vi "Create_Trajectory_Get_RectRegion_Constraint.vi"(11 "inTRAJECTORY_CONFIG":T1 {"End Velocity" format="%20.4f"; "StartVelocity" format="%20.4f"; "Max Acceleration" format="%20.4f"; "MaxVelocity" format="%20.4f"}) -> (1 "Constraint Exists":bool, 3 "Rect Region Constraint":T2={"BottomLeftPoint"={"X"=0.0, "Y"=0.0}, "TopRightPoint"={"X"=0.0, "Y"=0.0}, "Constraint"=variant, "Constraint Type"=enum."DIFF DRIVE KINEMATICS"} {"TopRightPoint"."Y" format="%14.3f"; "TopRightPoint"."X" format="%14.3f"; "BottomLeftPoint"."Y" format="%14.3f"; "BottomLeftPoint"."X" format="%14.3f"})   [LabVIEW 2019]
doc: "Retrieves the Differntial Drive Kinematics constraint from the Trajectory Configuration.\n\nNote: If more than once instance of the Differntial Drive Kinematics constraint exists only the first one is returned. (Only one of these should be defined.)\n\nParameters:\n - InTrajectoryConfig -- The trajectory configuration data structure\n\nReturns:\n - Diff Drive Kinematics Constraint -- The data cluster, which contains the constraint.\n - Constraint Exists -- Returns TRUE if this constraint is defined in the trjaectory configuration."
uses:
  <vilib>/Rock Robotics/WPI/ThirdParty/JAS_Junk/TrajLib/TypeDef/TRAJ_CONSTRAINT_RECT_REGION.ctl
  <vilib>/Rock Robotics/WPI/ThirdParty/JAS_Junk/TrajLib/TypeDef/TRANSLATION2D.ctl
  <vilib>/Rock Robotics/WPI/ThirdParty/JAS_Junk/TrajLib/Enum/TRAJ_CONSTRAINT_TYPES_ENUM.ctl
  <vilib>/Rock Robotics/WPI/ThirdParty/JAS_Junk/TrajLib/TypeDef/TRAJ_CONFIG.ctl
  <vilib>/Utility/Data Type/NI_Data Type.lvlib
  <vilib>/Rock Robotics/WPI/ThirdParty/JAS_Junk/TrajLib/Trajectory_Library.lvlib
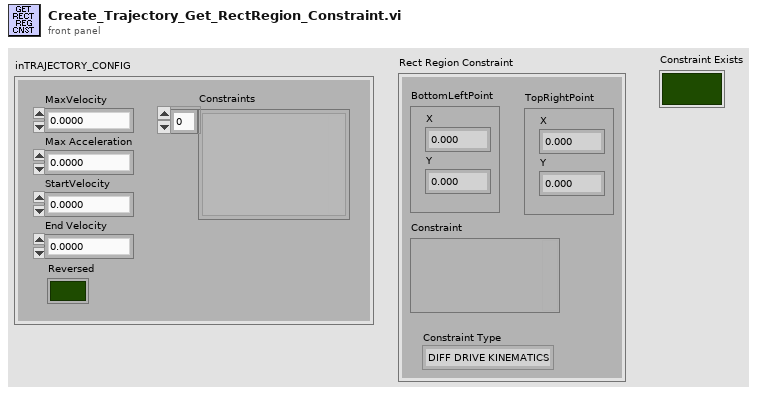
[diagram p1: front panel]
types:
  T1 = typedef "Trajectory_Library.lvlib/TRAJ_CONFIG.ctl" = cluster{"MaxVelocity":dbl, "Max Acceleration":dbl, "StartVelocity":dbl, "End Velocity":dbl, "Reversed":bool, "Constraints":variant[]}
  T2 = typedef "Trajectory_Library.lvlib/TRAJ_CONSTRAINT_RECT_REGION.ctl" = cluster{"BottomLeftPoint":T3, "TopRightPoint":T3, "Constraint":variant, "Constraint Type":T4}
  T3 = typedef "Trajectory_Library.lvlib/TRANSLATION2D.ctl" = cluster{"X":dbl, "Y":dbl}
  T4 = typedef "Trajectory_Library.lvlib/TRAJ_CONSTRAINT_TYPES_ENUM.ctl" = enum16{"UNDEFINED", "DIFF DRIVE KINEMATICS", "DIFF DRIVE VOLTAGE", "CENTRIPITAL ACCEL", "MECA DRIVE KINEMATICS", "SWERVE DRIVE KINEMATICS", "MAXIMUM VELOCITY", "ELLIPTICAL REGION", "RECTANGULAR REGION"}
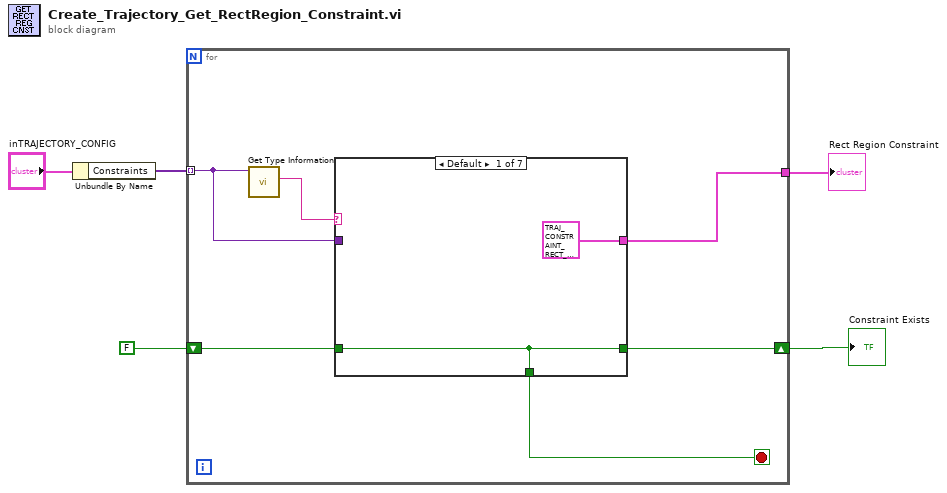
[diagram p0: block diagram]
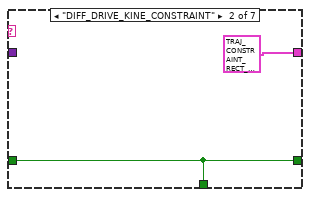
[diagram p2: hidden frame]
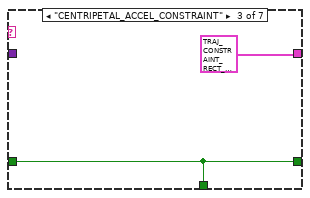
[diagram p3: hidden frame]
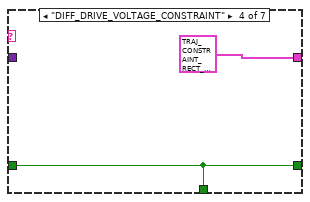
[diagram p4: hidden frame]
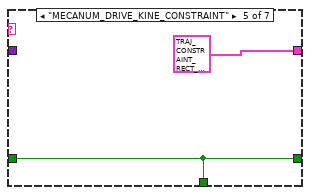
[diagram p5: hidden frame]
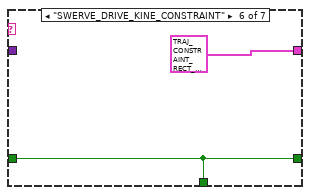
[diagram p6: hidden frame]
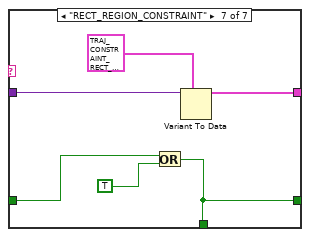
[diagram p7: hidden frame]
diagram:
  n1 = Unbundle By Name("inTRAJECTORY_CONFIG") -> ("Constraints"=w4:variant[])
  n2 = for {
    tunnel: w4 -> [w10] mode=indexing
    shift-right: [w8] -> w2
    shift-left: FALSE -> [w9]
    tunnel: [w6] -> w1
    stop <- w7 stop-if-true
    n3 = call <vilib>:"Get Type Information.vi"("variant"=w10) -> ("name"=w11:string)  [unwired: 6 in, 4 out]
    n4 = case shown="Default" w11 {
      tunnel: w10 -> [_ _ _ _ _ _ w25]
      tunnel: w9 -> [w13 w14 w17 w19 w21 w23 w28]
      tunnel: [w13 w14 w17 w19 w21 w23 w27] -> w8
      tunnel: [w13 w14 w17 w19 w21 w23 w27] -> w7
      tunnel: [T2 {"BottomLeftPoint"={"X"=0.0, "Y"=0.0}, "TopRightPoint"={"X"=0.0, "Y"=0.0}, "Constraint"=variant, "Constraint Type"=enum."DIFF DRIVE KINEMATICS"} ("Diff Drive Kinematics Constraint 2") T2 {"BottomLeftPoint"={"X"=0.0, "Y"=0.0}, "TopRightPoint"={"X"=0.0, "Y"=0.0}, "Constraint"=variant, "Constraint Type"=enum."DIFF DRIVE KINEMATICS"} ("Diff Drive Kinematics Constraint 2") T2 {"BottomLeftPoint"={"X"=0.0, "Y"=0.0}, "TopRightPoint"={"X"=0.0, "Y"=0.0}, "Constraint"=variant, "Constraint Type"=enum."DIFF DRIVE KINEMATICS"} ("Diff Drive Kinematics Constraint 2") T2 {"BottomLeftPoint"={"X"=0.0, "Y"=0.0}, "TopRightPoint"={"X"=0.0, "Y"=0.0}, "Constraint"=variant, "Constraint Type"=enum."DIFF DRIVE KINEMATICS"} ("Diff Drive Kinematics Constraint 2") T2 {"BottomLeftPoint"={"X"=0.0, "Y"=0.0}, "TopRightPoint"={"X"=0.0, "Y"=0.0}, "Constraint"=variant, "Constraint Type"=enum."DIFF DRIVE KINEMATICS"} ("Diff Drive Kinematics Constraint 2") T2 {"BottomLeftPoint"={"X"=0.0, "Y"=0.0}, "TopRightPoint"={"X"=0.0, "Y"=0.0}, "Constraint"=variant, "Constraint Type"=enum."DIFF DRIVE KINEMATICS"} ("Diff Drive Kinematics Constraint 2") w24] -> w6
      frame Default {
      }
      frame "DIFF_DRIVE_KINE_CONSTRAINT" {
      }
      frame "CENTRIPETAL_ACCEL_CONSTRAINT" {
      }
      frame "DIFF_DRIVE_VOLTAGE_CONSTRAINT" {
      }
      frame "MECANUM_DRIVE_KINE_CONSTRAINT" {
      }
      frame "SWERVE_DRIVE_KINE_CONSTRAINT" {
      }
      frame "RECT_REGION_CONSTRAINT" {
        n5 = Or(x=w28, y=TRUE) -> (x .or. y?=w27:bool)
        n6 = Variant To Data(type=T2 {"BottomLeftPoint"={"X"=0.0, "Y"=0.0}, "TopRightPoint"={"X"=0.0, "Y"=0.0}, "Constraint"=variant, "Constraint Type"=enum."DIFF DRIVE KINEMATICS"} ("Diff Drive Kinematics Constraint 2"), Variant=w25) -> (data=w24:T2)  [unwired: 1 in, 1 out]
      }
    }
  }
  "Rect Region Constraint" <- w1
  "Constraint Exists" <- w2
